vi "Load configuration.vi"(8 "error in":errorcluster, 11 "Path":path) -> (0 "error out":errorcluster, 3 "Configuration":T1)   [LabVIEW 2014]
uses:
  Configuration.ctl
  <vilib>/xml/Load XML File.vi
  <vilib>/xml/Close Reference(Node).vi
  <vilib>/xml/NI_XML.lvlib
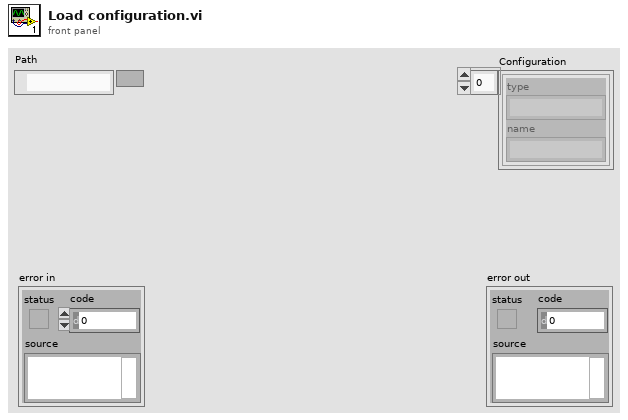
[diagram p1: front panel]
types:
  T1 = typedef "Configuration.ctl" = cluster{"type":string, "name":string}[]
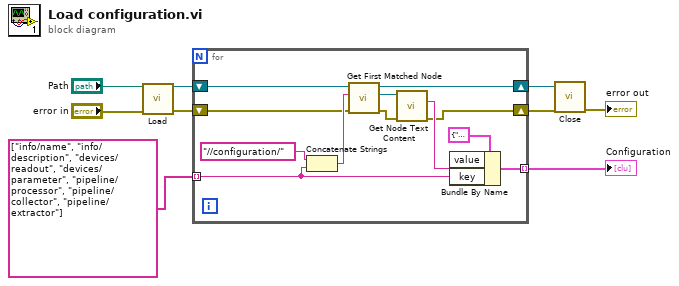
[diagram p0: block diagram]
diagram:
  n1 = call-poly <vilib>:"Load.vi"("path to XML document"="Path", "error in (no error)"="error in") -> ("DOM document out"=w8:refnum<k20>, "error out"=w6:errorcluster)  [unwired: 11 in, 1 out]
  n2 = for {
    tunnel: string[] ["info/name", "info/description", "devices/readout", "devices/parameter", "pipeline/processor", "pipeline/collector", "pipeline/extractor"] -> [w20] mode=indexing
    shift-right: [w17] -> w7
    shift-left: w8 -> [w18]
    tunnel: [w19] -> w4 mode=indexing
    shift-right: [w10] -> w5
    shift-left: w6 -> [w12]
    n3 = Concatenate Strings("//configuration/", w20) -> (w16:string)
    n4 = call <vilib>:"Get First Matched Node.vi"("error in (no error)"=w12, "XPath expression"=w16, "node in"=w18) -> ("error out"=w11:errorcluster, "node result"=w14:refnum<k20>, "node out"=w17:refnum<k20>)  [unwired: 6 in]
    n5 = call <vilib>:"Get Node Text Content.vi"("error in (no error)"=w11, "node in"=w14) -> ("error out"=w10:errorcluster, "node text"=w13:string)  [unwired: 7 in, 1 out]
    n6 = Bundle By Name(cluster=cluster{"key":string, "value":string} {"key"="", "value"=""}, "value"=w13, "key"=w20) -> (w19:cluster{"key":string, "value":string})
  }
  "Configuration" <- w4
  n7 = call-poly <vilib>:"Close.vi"("error in (no error)"=w5, "node"=w7) -> ("error out"=→"error out":errorcluster)  [unwired: 7 in]
